vi "send interpolated data.vi"(8 "error in (no error)":errorcluster, 9 "binary array":dbl[](array[numeric]), 10 "Interpolated data":dbl[][](array[numeric]), 11 "Autofocus in":refnum<class "Autofocus.lvclass">) -> (0 "error out":errorcluster, 3 "Autofocus out":refnum<class "Autofocus.lvclass">)   [LabVIEW 2012, in "Autofocus.lvclass"]
uses:
  Autofocus.lvclass
  <vilib>/Distrio/Murmex/Murmex/Murmex.lvclass
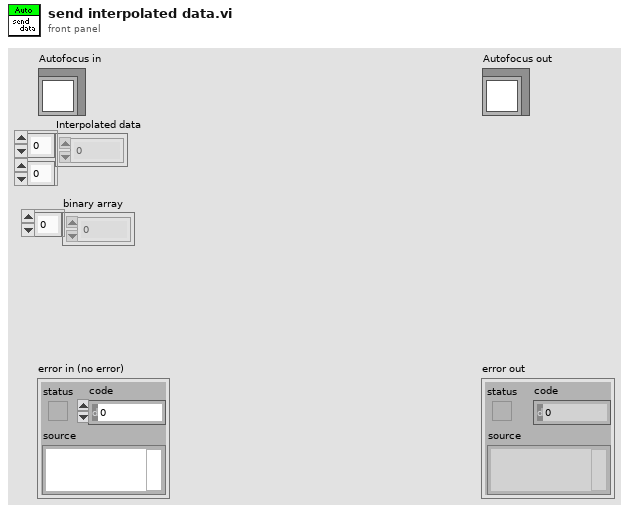
[diagram p1: front panel]
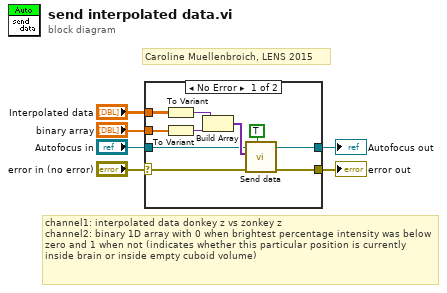
[diagram p0: block diagram]
diagram:
  # "channel1: interpolated data donkey z vs zonkey z\nchannel2: binary 1D array with 0 when brightest percentage intensity was below zero and 1 when not (indicates whether this particular position is currently inside brain or inside empty cuboid volume)"
  # "Caroline Muellenbroich, LENS 2015"
  n1 = case shown="No Error" "error in (no error)" {
    selector: "error in (no error)" -> [w14 w18]
    tunnel: [w13 w18] -> w5
    tunnel: [w11 w17] -> w3
    tunnel: "Autofocus in" -> [w12 w17]
    tunnel: "Interpolated data" -> [w8 _]
    tunnel: "binary array" -> [w7 _]
    frame No Error {
      n2 = To Variant(anything=w8) -> (Variant=w10:variant)
      n3 = To Variant(anything=w7) -> (Variant=w9:variant)
      n4 = Build Array(w10, w9) -> (w15:variant[])
      n5 = call <vilib>:"Send data.vi"("is finalised data? (T)"=TRUE, "error in (no error)"=w14, "data (channels array)"=w15, "Murmex in"=w12) -> ("error out"=w13:errorcluster, "Murmex out"=w11:refnum<class "Autofocus.lvclass">)  [unwired: 6 in]
    }
    frame Error {
    }
  }
  "error out" <- w5
  "Autofocus out" <- w3
